vi "Acquisition_a.vi"() -> (4 "Acquired_Data":dbl(graph))   [LabVIEW 2023]
doc: "This VI acquire data that were generated be the Generator VI.\nTransfer of thet data happens under Global variable."
uses:
  Global_Variables/Generate_Data_Global.vi
panel:
  out "Error_Out":errorcluster
  in  "Error_In":errorcluster
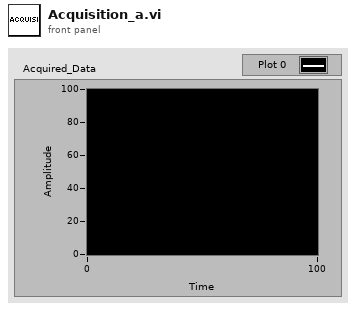
[diagram p1: front panel]
types:
  T1 = enum16{"Left Button", "Center Button", "Right Button", "Window Close"}
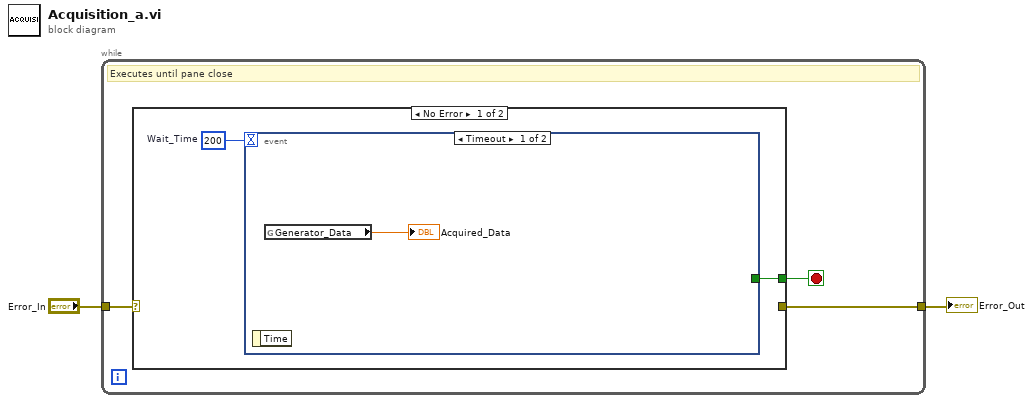
[diagram p0: block diagram]
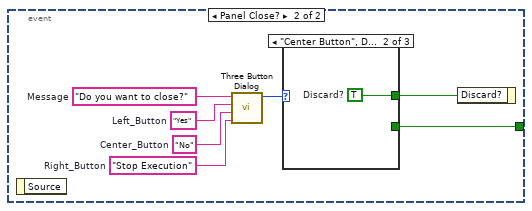
[diagram p2: hidden frame]
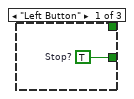
[diagram p3: hidden frame]
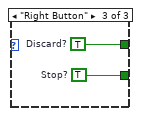
[diagram p4: hidden frame]
diagram:
  n1 = while {
    tunnel: "Error_In" -> [w4]
    tunnel: [w3] -> w1
    stop <- w5 stop-if-true
    # "Executes until pane close"
    n2 = case shown="No Error" w4 {
      selector: w4 -> [_ w20]
      tunnel: [w6 _] -> w5
      tunnel: [_ w20] -> w3
      frame No Error {
        w7 = 200  # Wait_Time
        n3 = event shown="[0] Timeout" {
          selector: _ -> [_ _]
          dyn-events: _ -> [_ _]
          timeout: w7 -> [_ _]
          tunnel: [_ w9] -> w6
          event Timeout {
            n4 = event-data() -> ()  [unwired: 1 in, 1 out]
            n5 = global read "Generate_Data_Global.vi" "Generator_Data"() -> (→"Acquired_Data":dbl)
          }
          event Panel Close? {
            w12 = "Stop Execution"  # Right_Button
            w13 = "No"  # Center_Button
            w14 = "Yes"  # Left_Button
            w15 = "Do you want to close?"  # Message
            n6 = event-data() -> ()  [unwired: 1 in, 1 out]
            n7 = call <vilib>:"Three Button Dialog.vi"("Right Button Text (\"Cancel\")"=w12, "Center Button Text (\"No\")"=w13, "Left Button Text (\"Yes\")"=w14, "message"=w15) -> ("Which Button?"=w11:T1)  [unwired: 7 in]
            n8 = case shown="\"Center Button\", Default" w11 {
              tunnel: [_ w17 w18] -> w10
              tunnel: [w16 _ w19] -> w9
              frame "Left Button" {
                w16 = TRUE  # Stop?
              }
              frame "Center Button", Default {
                w17 = TRUE  # Discard?
              }
              frame "Right Button" {
                w18 = TRUE  # Discard?
                w19 = TRUE  # Stop?
              }
            }
            n9 = event-data("Discard?"=w10) -> ()  [unwired: 1 in, 1 out]
          }
        }
      }
      frame Error {
      }
    }
  }
  "Error_Out" <- w1
